vi "OAT Filtered Orbit Plot.vi"(0 "magnitudes":cluster{"X":dbl[], "Y":dbl[]}[](array[cluster]) {"Y" format="%.2f"; "X" format="%.2f"}, 1 "XY graph Ref":refnum<vi>, 2 "order":dbl=1.0 format="%.2f", 5 "phase lags":cluster{"X":dbl[], "Y":dbl[]}[](array[cluster]) {"Y" format="%.2f"; "X" format="%.2f"}, 7 "samples/rev":dbl=1.0 format="%.2f", 9 "samples/rev wanted":i32=64, 11 "error in (no error)":errorcluster, 12 "orbit segment":cluster{"position":dbl, "tach duty":dbl}={"position"=0.0, "tach duty"=0.98} {"tach duty" format="%.2f"; "position" format="%.2f"}, 13 "phase setting":T1, 14 "probe angle":u16(ring) items=["0", "45", "90", "135", "180", "225", "270", "315"]) -> (4 "XY plot value":cluster{"X":dbl[], "Y":dbl[]}[](array[cluster]) {"Y" format="%.2f"; "X" format="%.2f"}, 15 "error out":errorcluster)   [LabVIEW 2017]
doc: "Draws an orbit plot of magnitude and phase data on a XY graph."
uses:
  <vilib>/addons/Sound and Vibration/Order Analysis/Resample Order Tracking/SoundVib_Resampling.lvlib
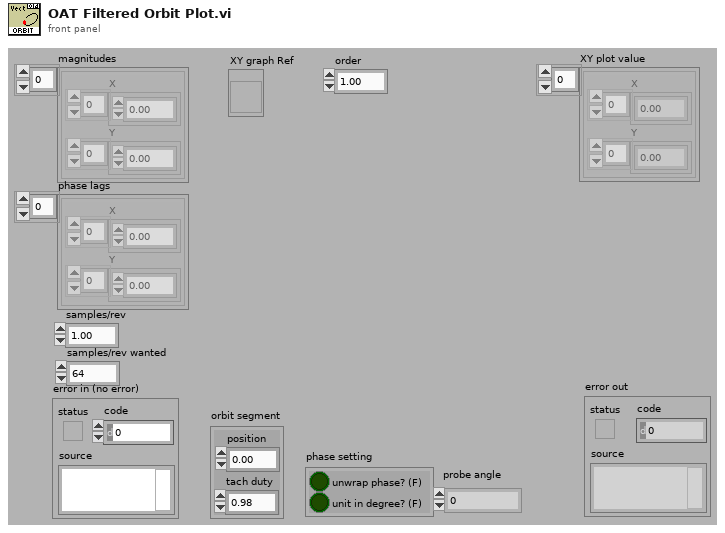
[diagram p1: front panel]
types:
  T1 = cluster{"unwrap phase? (F)":bool, "unit in degree? (F)":bool}
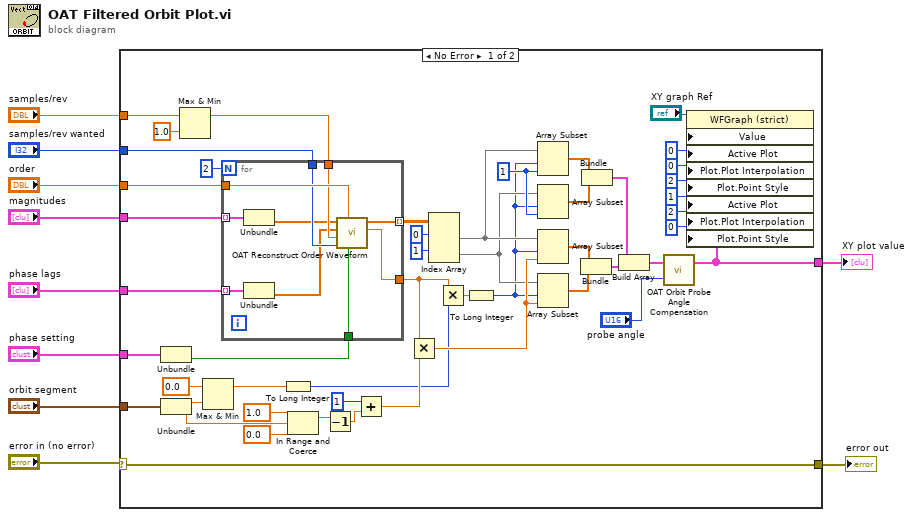
[diagram p0: block diagram]
diagram:
  n1 = case shown="No Error" "error in (no error)" {
    selector: "error in (no error)" -> [w17 w70]
    tunnel: "order" -> [w54 _]
    tunnel: "samples/rev wanted" -> [w53 _]
    tunnel: "magnitudes" -> [w51 _]
    tunnel: "phase lags" -> [w50 _]
    tunnel: "phase setting" -> [w42 _]
    tunnel: "orbit segment" -> [w40 _]
    tunnel: "samples/rev" -> [w13 _]
    tunnel: [w16 _] -> w3
    tunnel: [w17 w70] -> w1
    frame No Error {
      w57 = 1 ("length")
      n2 = Unbundle(w42) -> ("unit in degree? (F)"=w41:bool)  [unwired: 1 out]
      n3 = Unbundle(w40) -> ("position"=w21:dbl, "tach duty"=w24:dbl)
      n4 = Max & Min(x=w13, y=1.0) -> (max(x,y)=w12:dbl)  [unwired: 1 out]
      n5 = Max & Min(x=0.0 ("t"), y=w21) -> (max(x,y)=w20:dbl)  [unwired: 1 out]
      n6 = for {
        N: 2 -> [_]
        tunnel: [w69] -> w47 mode=indexing
        tunnel: w54 -> [w68]
        tunnel: w53 -> [w67]
        tunnel: w12 -> [w66]
        tunnel: w51 -> [w65] mode=indexing
        tunnel: w50 -> [w64] mode=indexing
        tunnel: [w60] -> w39
        tunnel: w41 -> [w63]
        n7 = Unbundle(w65) -> ("Y"=w62:dbl[])  [unwired: 1 out]
        n8 = Unbundle(w64) -> ("Y"=w61:dbl[])  [unwired: 1 out]
        n9 = call <vilib>:"OAT Reconstruct Order Waveform.vi"("unit in degree? (F)"=w63, "order"=w68, "samples/revolution wanted"=w67, "samples/revolution"=w66, "phase lag"=w61, "magnitude"=w62) -> ("actual samples/rev"=w60:dbl, "order waveform"=w69:dbl[])  [unwired: 3 in, 1 out]
      }
      n10 = To Long Integer(number=w20) -> (32bit integer=w19:i32)
      n11 = In Range and Coerce(upper limit=1.0, x=w24, lower limit=0.0 ("upper limit")) -> (coerced(x)=w26:dbl)  [unwired: 1 out]
      n12 = Decrement(x=w26) -> (x-1=w25:dbl)
      n13 = Add(x=1 ("t"), y=w25) -> (x+y=w29:dbl)
      n14 = Multiply(x=w39, y=w29) -> (x*y=w45:dbl)
      n15 = Index Array(array=w47, index (row) #1=0 ("index (row)"), index (row) #2=1 ("index (row)")) -> (element #1=w44:dbl[], element #2=w30:dbl[])  [unwired: 2 in]
      n16 = Multiply(x=w39, y=w19) -> (x*y=w38:dbl)
      n17 = To Long Integer(number=w38) -> (32bit integer=w18:i32)
      n18 = Array Subset(array=w44, index=w18, length=w57) -> (w59:dbl[])
      n19 = Array Subset(array=w30, index=w18, length=w57) -> (w58:dbl[])
      n20 = Array Subset(array=w44, index=w18, length=w45) -> (w43:dbl[])
      n21 = Array Subset(array=w30, index=w18, length=w45) -> (w46:dbl[])
      n22 = Bundle(w43, w46) -> (w55:cluster{dbl[], dbl[]})  [unwired: 1 in]
      n23 = Bundle(w59, w58) -> (w56:cluster{dbl[], dbl[]})  [unwired: 1 in]
      n24 = Build Array(w56, w55) -> (w14:cluster{dbl[], dbl[]}[])
      n25 = call <vilib>:"OAT Orbit Probe Angle Compensation.vi"("probe angle compensation"="probe angle", "XY plot data in"=w14) -> ("XY plot data out"=w16:cluster{dbl[], dbl[]}[])  [unwired: 1 in]
      n26 = property class="WFGraph (strict)"(reference="XY graph Ref", "Value"=w16, "Active Plot"=u32 0, "Plot.Plot Interpolation"=u8 0, "Plot.Point Style"=u8 2, "Active Plot"=u32 1, "Plot.Plot Interpolation"=u8 2, "Plot.Point Style"=u8 0) -> ()  [unwired: 1 in, 2 out]
    }
    frame Error {
    }
  }
  "XY plot value" <- w3
  "error out" <- w1
